vi "Pre Launch Init.vi"(11 "IModel in":refnum<class "IModel.lvclass">) -> (0 "error out":errorcluster, 3 "IModel out":refnum<class "IModel.lvclass">)   [LabVIEW 2015, in "IModel.lvlib" / "IModel.lvclass"]
doc: "(<B>Filename</B>: Actor Framework.lvlib:Actor.lvclass:Pre Launch Init.vi)\n\nDefines behavior that occurs after the Launch Nested Actor method is invoked but before the actor's Actor Core method begins running.\n\nBy default, this method does nothing. A descendant class may override it to define behavior."
uses:
  IModel.lvclass
  <vilib>/ActorFramework/Actor/Actor.lvclass/Actor.ctl
  <vilib>/ActorFramework/Message Enqueuer/Message Enqueuer.lvclass/Message Enqueuer.ctl
  IModel.lvclass/IModel.ctl
  <vilib>/ActorFramework/Message Enqueuer/Init from Existing Queue.vi
  <vilib>/ActorFramework/Actor/Actor.lvclass
  <vilib>/ActorFramework/Message Enqueuer/Message Enqueuer.lvclass
  IModel Messages/Launch Nested Models Msg/Launch Nested Models Msg.lvclass
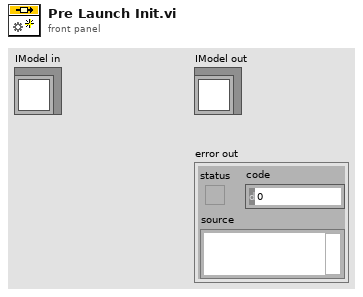
[diagram p1: front panel]
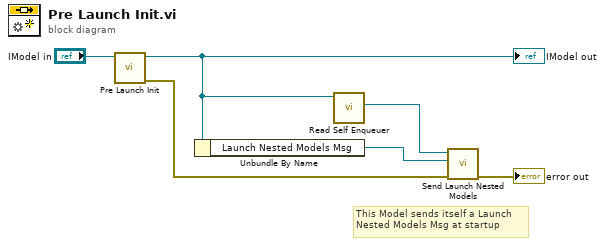
[diagram p0: block diagram]
diagram:
  # "This Model sends itself a Launch\nNested Models Msg at startup"
  n1 = call-parent "Pre Launch Init.vi"("Actor in"="IModel in") -> ("error out"=w4:errorcluster, "Actor out"=w2:refnum<class "IModel.lvclass">)  [unwired: 9 in]
  "IModel out" <- w2
  n2 = Unbundle By Name(w2) -> ("Launch Nested Models Msg"=w1:refnum<class "Launch Nested Models Msg.lvclass">)
  n3 = call <vilib>:"Read Self Enqueuer.vi"("Actor"=w2) -> ("Self Enqueuer"=w5:refnum<class "Message Enqueuer.lvclass">)  [unwired: 10 in]
  n4 = call-dynamic "Send Launch Nested Models.vi"("error in (no error)"=w4, "Launch Nested Models Msg"=w1, "Message Enqueuer"=w5) -> ("error out"=→"error out":errorcluster)  [unwired: 7 in, 1 out]
